vi "LHF.DB.Mongo.Util.BuildConnectionString.vi"(0 "host":string="localhost", 1 "port":u32=27017) -> (14 "connectionString":string="mongodb://localhost:27017/")   [LabVIEW 2013, in "LHF.DB.Mongo.lvclass"]
uses:
  LHF.DB.Mongo.lvclass
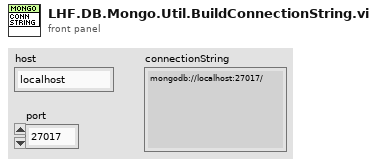
[diagram p1: front panel]
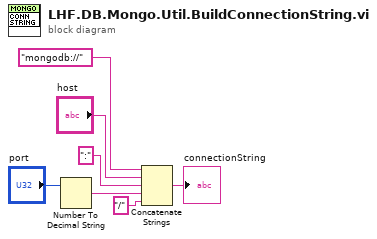
[diagram p0: block diagram]
diagram:
  n1 = Number To Decimal String(number="port") -> (decimal integer string=w2:string)  [unwired: 1 in]
  n2 = Concatenate Strings("mongodb://" ("connectionString"), "host", ":" ("string"), w2, "/" ("string")) -> (→"connectionString":string)
